vi "Read Measure.vi"(0 "VISA resource name":refnum<visa-resource-name>, 11 "error in (no error)":errorcluster) -> (4 "VISA resource name out":refnum<visa-resource-name>, 6 "Read Strings":string, 8 "Measure Value":sgl[](array[numeric]) format="%^.3e", 15 "error out":errorcluster)   [LabVIEW 2013, in "Yokogawa WT200 Series.lvlib"]
doc: "This VI reads the Measure Value from the WT200 Series."
uses:
  <instrlib>/Yokogawa WT200 Series/Yokogawa WT200 Series.lvlib
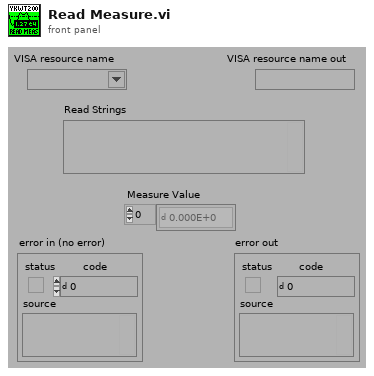
[diagram p1: front panel]
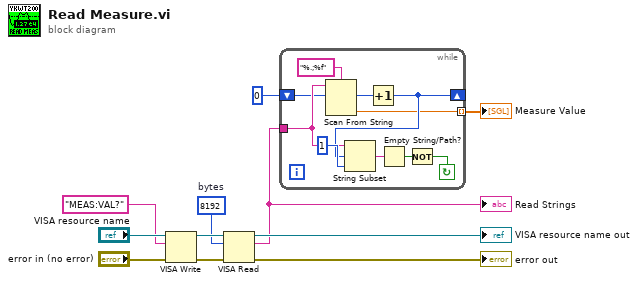
[diagram p0: block diagram]
diagram:
  w1 = u32 8192  # bytes
  n1 = VISA Write(VISA resource name="VISA resource name", write buffer="MEAS:VAL?", error in (no error)="error in (no error)") -> (VISA resource name out=w7:refnum<visa-resource-name>, error out=w8:errorcluster)  [unwired: 1 out]
  n2 = VISA Read(VISA resource name=w7, byte count=w1, error in (no error)=w8) -> (VISA resource name out=→"VISA resource name out":refnum<visa-resource-name>, read buffer=w3:string, error out=→"error out":errorcluster)  [unwired: 1 out]
  "Read Strings" <- w3
  n3 = while {
    tunnel: [w14] -> w2 mode=indexing
    shift-left: u32 0 -> [w15]
    shift-right: [w17] -> _
    tunnel: w3 -> [w16]
    stop <- w18 continue-if-true
    n4 = Scan From String(format string="%.;%f", input string=w16, initial scan location=w15) -> (offset past scan=w13:u32, output 1=w14:dbl)  [unwired: 2 in, 2 out]
    n5 = Increment(x=w13) -> (x+1=w17:u32)
    n6 = String Subset(string=w16, offset (0)=w17, length (rest)=1) -> (substring=w20:string)
    n7 = Empty String/Path?(string/path=w20) -> (empty?=w19:bool)
    n8 = Not(x=w19) -> (.not. x?=w18:bool)
  }
  "Measure Value" <- w2
